vi "Draw Body.vi"(8 "error in":errorcluster, 9 "Image":T2, 10 "Body Data":T3[](array[typedef]) {"LeanTrackingState" items=["NotTracked", "Inferred", "Tracked"]; "HandRightState" items=["Unknown", "NotTracked", "Open", "Closed", "Lasso"]; "HandRightConfidence" items=["Low", "High"]; "HandLeftState" items=["Unknown", "NotTracked", "Open", "Closed", "Lasso"]; "HandLeftConfidence" items=["Low", "High"]; "ClippedEdges" items=["None"=0, "Right"=1, "Left"=2, "Top"=4, "Bottom"=8]}, 11 "KinectSensor References":T1) -> (0 "error out":errorcluster, 1 "Image Out":T2, 3 "KinectSensor References out":T1)   [LabVIEW 2014]
uses:
  controls/BodyData.ctl
  Microsoft.Kinect
  controls/KinectSensor References.ctl
  C:/Users/iknox/Documents/BodyFrameDataInterface/bin/Debug/BodyFrameDataInterface.dll
  Users/iknox/Documents/BodyFrameDataInterface/bin/Debug/BodyFrameDataInterface.dll
  <vilib>/vision/Image Controls.llb/IMAQ Image.ctl
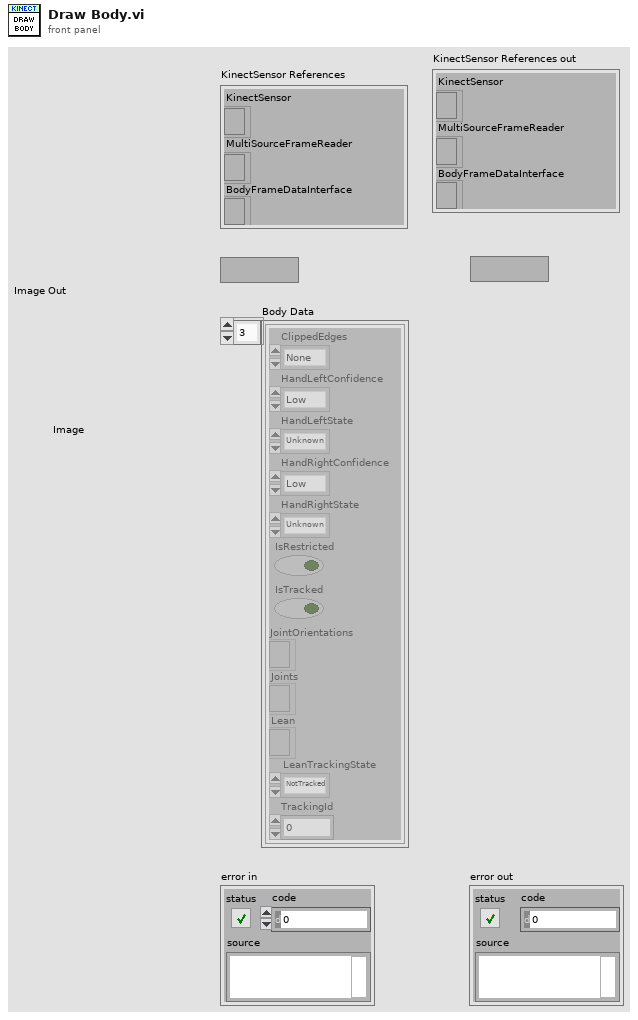
[diagram p1: front panel]
types:
  T1 = typedef "KinectSensor References.ctl" = cluster{"KinectSensor":refnum<k24>, "MultiSourceFrameReader":refnum<k24>, "BodyFrameDataInterface":refnum<k24>}
  T2 = typedef "IMAQ Image.ctl" = refnum<image>
  T3 = typedef "BodyData.ctl" = cluster{"ClippedEdges":i32, "HandLeftConfidence":i32, "HandLeftState":i32, "HandRightConfidence":i32, "HandRightState":i32, "IsRestricted":bool, "IsTracked":bool, "JointOrientations":refnum<k24>, "Joints":refnum<k24>, "Lean":refnum<k24>, "LeanTrackingState":i32, "TrackingId":u64}
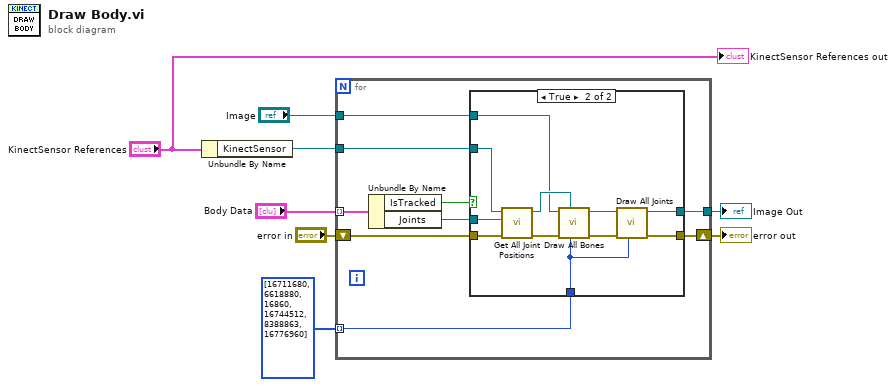
[diagram p0: block diagram]
diagram:
  n1 = Unbundle By Name("KinectSensor References") -> ("KinectSensor"=w6:refnum<k24>)
  n2 = for {
    tunnel: "Body Data" -> [w17] mode=indexing
    tunnel: w6 -> [w14]
    shift-right: [w13] -> w4
    shift-left: "error in" -> [w12]
    tunnel: "Image" -> [w11]
    tunnel: [w10] -> w2
    tunnel: u32[] [16711680, 6618880, 16860, 16744512, 8388863, 16776960] -> [w9] mode=indexing
    n3 = Unbundle By Name(w17) -> ("IsTracked"=w16:bool, "Joints"=w15:refnum<k24>)
    n4 = case shown="True" w16 {
      tunnel: w15 -> [_ w30]
      tunnel: w14 -> [_ w28]
      tunnel: [w19 w23] -> w13
      tunnel: w12 -> [w19 w27]
      tunnel: w11 -> [w18 w25]
      tunnel: [w18 w21] -> w10
      tunnel: w9 -> [_ w20]
      frame False {
      }
      frame True {
        n5 = call "Get All Joint Positions.vi"("error in (no error)"=w27, "Joints"=w30, "KinectSensor Reference"=w28) -> ("error out"=w29:errorcluster, "Joints"=w26:refnum<k24>)  [unwired: 7 in]
        n6 = call "Draw All Bones.vi"("Color"=w20, "Joints"=w26, "error in"=w29, "Image"=w25) -> ("error out"=w24:errorcluster, "Image Out"=w22:T2)  [unwired: 6 in]
        n7 = call "Draw All Joints.vi"("Color"=w20, "error out"=w24, "Image"=w22) -> ("error out 2"=w23:errorcluster, "Image Out"=w21:T2)  [unwired: 7 in]
      }
    }
  }
  "error out" <- w4
  "Image Out" <- w2
  "KinectSensor References out" <- "KinectSensor References"
